vi "WriteToDb.vi"(0 "reference in":refnum<class "Sig_AI.lvclass">, 11 "error in (no error)":errorcluster) -> (4 "reference out":refnum<class "Sig_AI.lvclass">, 15 "error out":errorcluster)   [LabVIEW 2019, in "Sig_AI.lvclass"]
uses:
  Sig_AI.lvclass
  D:/GIT H4000/H4000/src/Proccess_class/Proccess.lvclass
  Proccess_class/Proccess.lvclass/Proccess.ctl
  Sig_AI.lvclass/Sig_AI.ctl
  Logger_class/SignalData.ctl
  TypeDef/engineering units.ctl
  Logger_class/Logger.lvclass/Logger.ctl
  Logger_class/Logger.lvclass
  Proccess_class/Proccess.lvclass
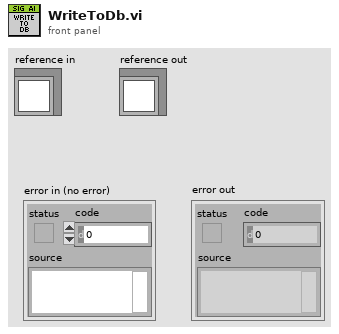
[diagram p1: front panel]
types:
  T1 = typedef "Logger.lvclass/SignalData.ctl" = cluster{"Value":dbl, "SignalTag":string, "ObjTag":string, "engineering units":T2, "Desc":string, "Time Stamp":timestamp}
  T2 = typedef "engineering units.ctl" = enum16{"mV", "V", "mA", "A", "C", "pC", "s", "Pa", "N", "g", "m/s^2", "m/s", "m", "mm/s", "mm", "micron/s", "micron", "in/s^2", "in/s", "in", "mil/s", "mil", "rad/s^2", "rad/s", "rad", "deg/s^2", "deg/s", "deg", "RPM", "cycle/s^2", "Hz", "cycle", "strain", "%"}
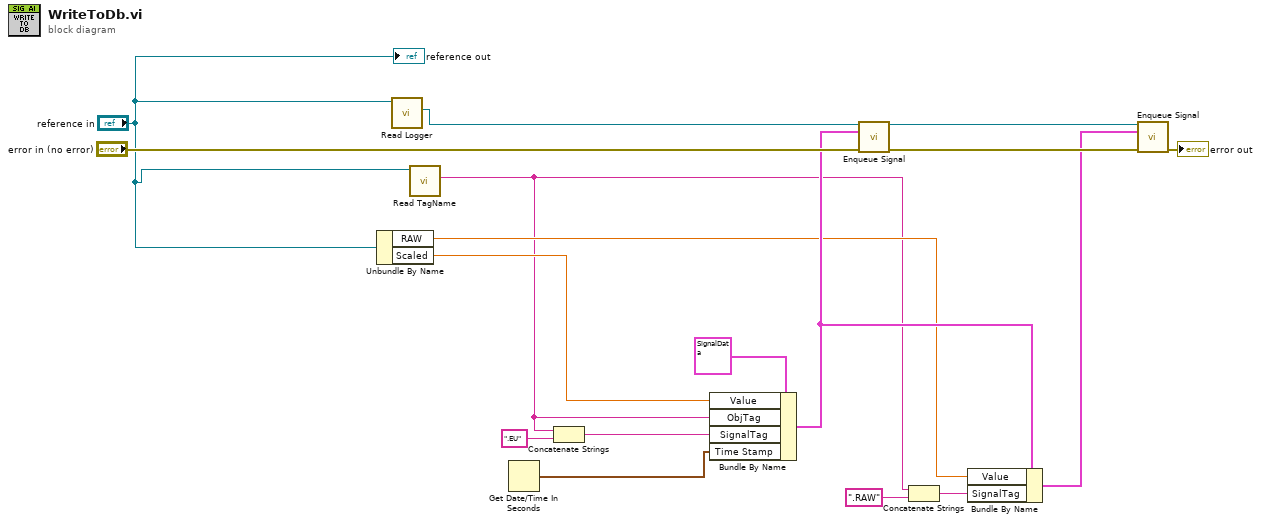
[diagram p0: block diagram]
diagram:
  n1 = Unbundle By Name("reference in") -> ("RAW"=w8:dbl, "Scaled"=w12:dbl)
  n2 = call "Read Logger.vi"("Proccess in"="reference in") -> ("Logger"=w2:refnum<class "Logger.lvclass">)  [unwired: 9 in, 1 out]
  n3 = call "Read TagName.vi"("Proccess in"="reference in") -> ("TagName"=w3:string)  [unwired: 9 in, 1 out]
  n4 = Get Date/Time In Seconds() -> (seconds since 1Jan1904=w14:timestamp)
  n5 = Concatenate Strings(w3, ".EU" ("string")) -> (w15:string)
  n6 = Bundle By Name(cluster=T1 {"Value"=0.0, "SignalTag"="", "ObjTag"="", "engineering units"=enum."A", "Desc"="", "Time Stamp"=timestamp(0 s since 1904-01-01)} ("element"), "Value"=w12, "ObjTag"=w3, "SignalTag"=w15, "Time Stamp"=w14) -> (w9:T1)
  n7 = call "Enqueue Signal.vi"("reference in"=w2, "element"=w9, "error in (no error)"="error in (no error)") -> ("reference out"=w11:refnum<class "Logger.lvclass">, "error out"=w10:errorcluster)  [unwired: 11 in]
  n8 = Concatenate Strings(w3, ".RAW" ("string")) -> (w6:string)
  n9 = Bundle By Name(cluster=w9, "Value"=w8, "SignalTag"=w6) -> (w5:T1)
  n10 = call "Enqueue Signal.vi"("reference in"=w11, "element"=w5, "error in (no error)"=w10) -> ("error out"=→"error out":errorcluster)  [unwired: 11 in, 1 out]
  "reference out" <- "reference in"
